vi "Loading Sequence.vi"(8 "Abort":bool, 9 "desired drop":dbl=8.0, 10 "Raised Tote Position":dbl=31.0, 11 "Button":bool) -> ()   [LabVIEW 2014]
uses:
  Loading States.ctl
  Robot Global Data.vi
  Desired Arm Position.vi
panel:
  out "Go all the way down":bool
  out "Wait for Unload":bool
  out "Lower Arms Slightly":bool
  out "Wait for Load":bool
  out "Raise Totes":bool
  out "Start + Wait for Totes":bool=TRUE
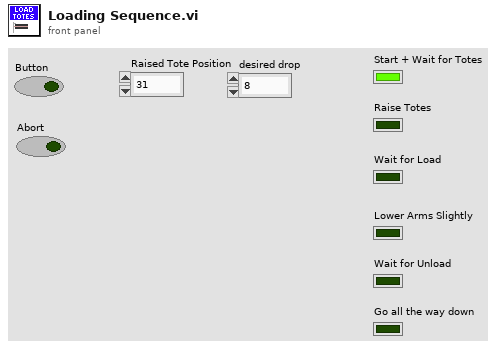
[diagram p1: front panel]
types:
  T1 = typedef "Loading States.ctl" = enum16{"Start+Wait for Totes", "Raise 2 Totes", "Wait for Loading", "Lower 2 Totes slightly", "Wait for Unload", "Go All the Way Down"}
  T2 = typedef "WPI_DigitalInputDevRef.ctl" = cluster{"DevStatus":errorcluster, "DIO Channel":T3, "Controller":T4}
  T3 = typedef "FPGA_DIOChannel.ctl" = enum8{"DIO 0", "DIO 1", "DIO 2", "DIO 3", "DIO 4", "DIO 5", "DIO 6", "DIO 7", "DIO 8", "DIO 9", "DIO MXP 0", "DIO MXP 1", "DIO MXP 2", "DIO MXP 3", "DIO MXP 4", "DIO MXP 5", "DIO MXP 6", "DIO MXP 7", "DIO MXP 8", "DIO MXP 9", "DIO MXP 10", "DIO MXP 11", "DIO MXP 12", "DIO MXP 13", "DIO MXP 14", "DIO MXP 15", "Invalid"}
  T4 = typedef "FPGA_TypedefDigitalModule.ctl" = enum16{"Controller 1"}
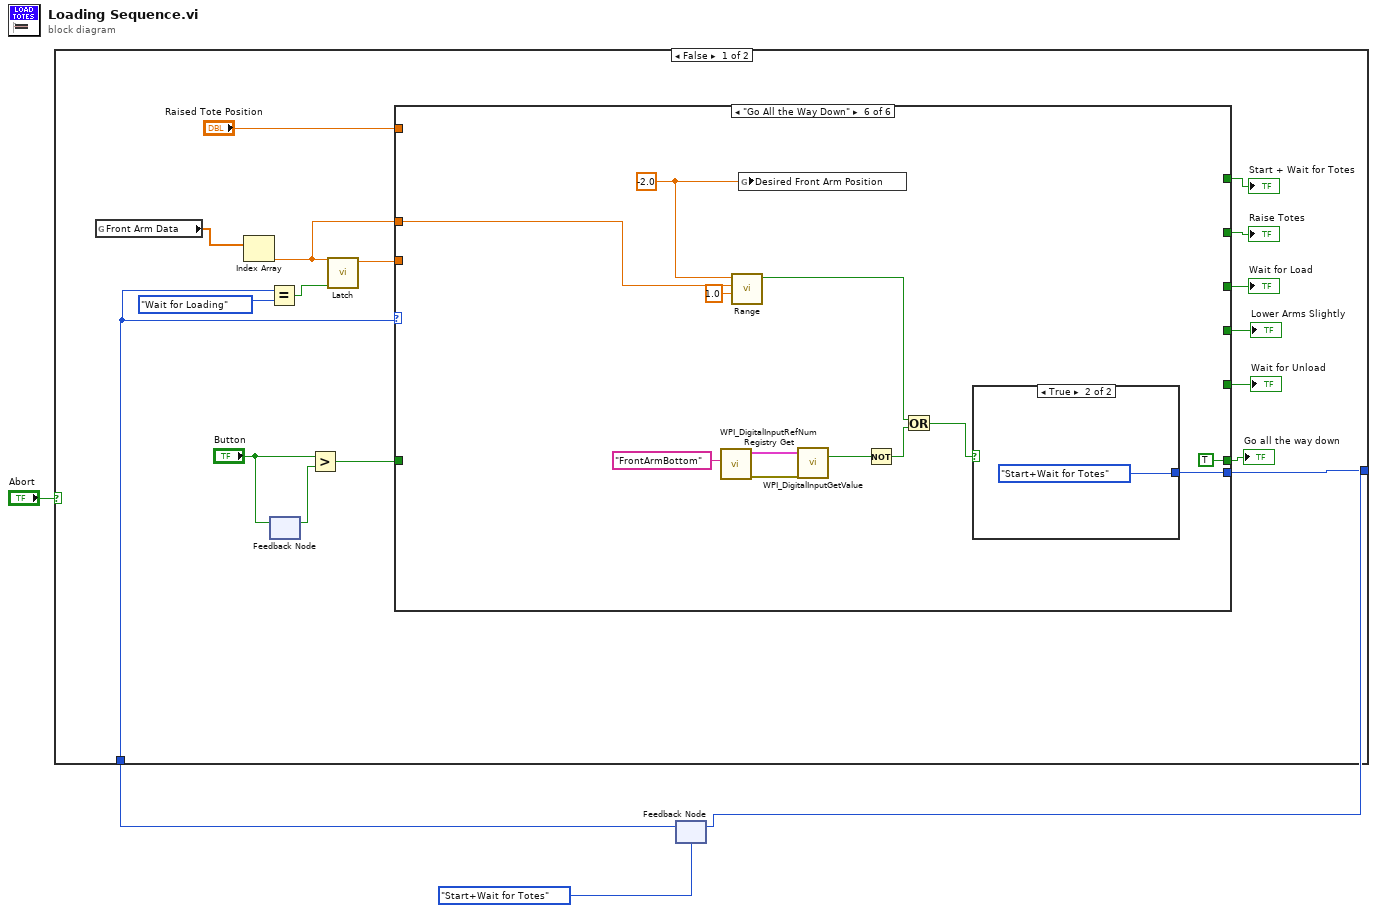
[diagram p0: block diagram]
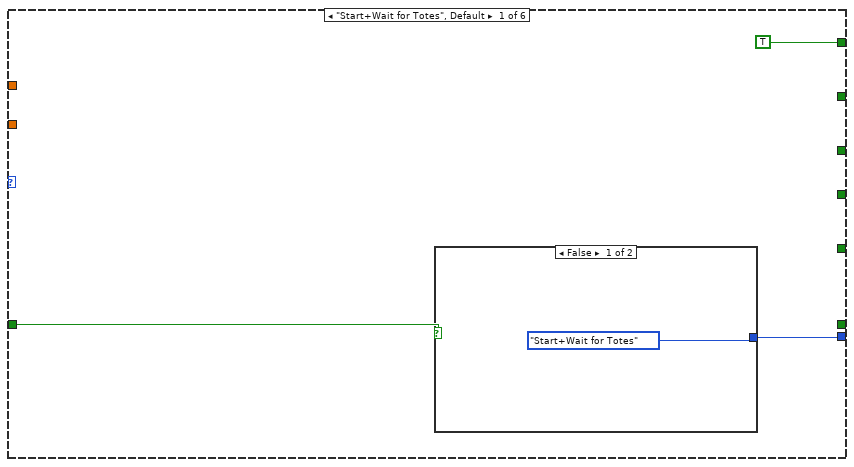
[diagram p2: hidden frame]
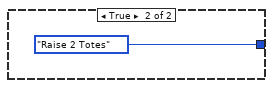
[diagram p3: hidden frame]
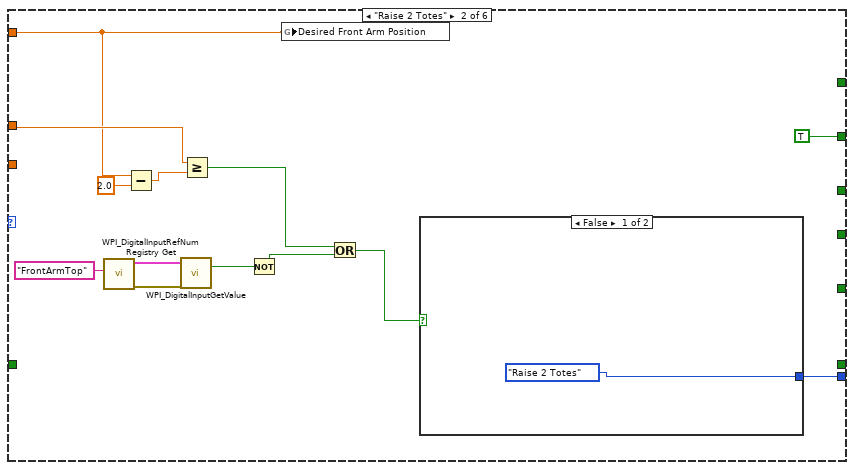
[diagram p4: hidden frame]
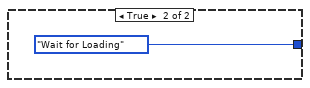
[diagram p5: hidden frame]
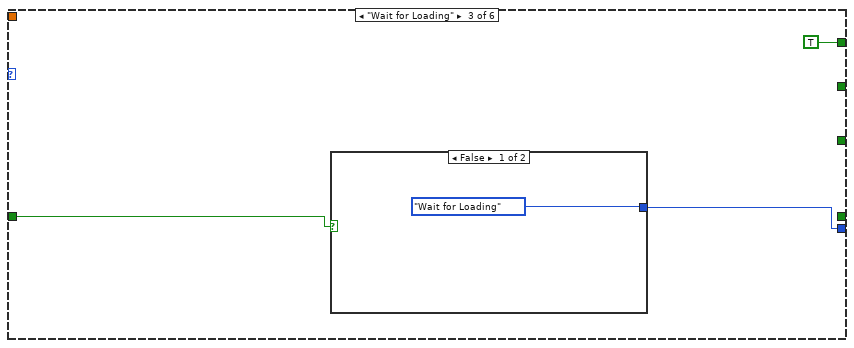
[diagram p6: hidden frame]
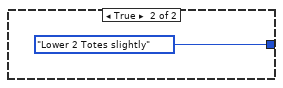
[diagram p7: hidden frame]
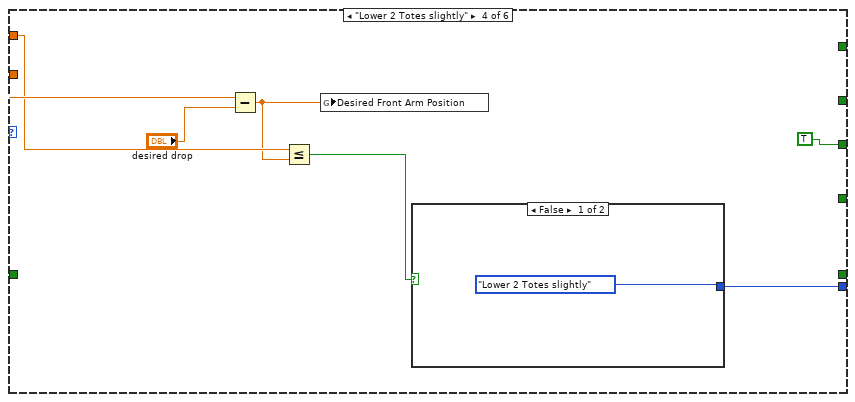
[diagram p8: hidden frame]
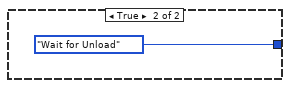
[diagram p9: hidden frame]
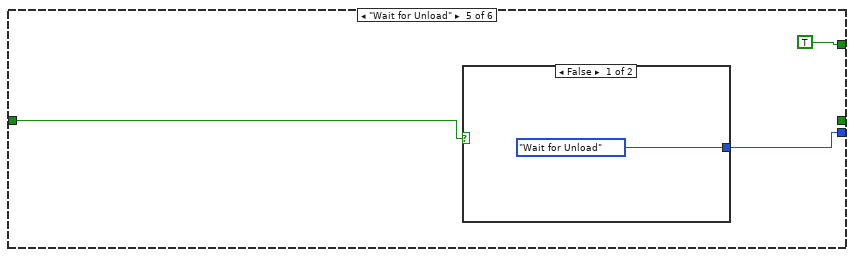
[diagram p10: hidden frame]
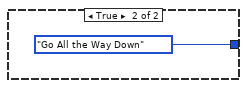
[diagram p11: hidden frame]
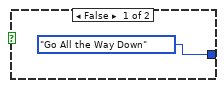
[diagram p12: hidden frame]
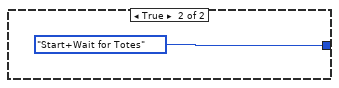
[diagram p13: hidden frame]
diagram:
  n1 = feedback #1(Loading_States."Start+Wait for Totes" ("Enum")) -> (w1:T1)
  n2 = case shown="False" "Abort" {
    tunnel: [w13 Loading_States."Start+Wait for Totes" ("Enum")] -> w2
    tunnel: w1 -> [w12 _]
    frame False {
      n3 = global read "Robot Global Data.vi" "Front Arm Data"() -> (w17:dbl[])
      n4 = Index Array(array=w17) -> (element=w5:dbl)  [unwired: 1 in]
      n5 = Equal?(x=w12, y=Loading_States."Wait for Loading" ("Enum")) -> (x = y?=w14:bool)
      n6 = feedback #2() -> (w20:bool)  [unwired: 1 in]
      n7 = feedback-in #2("Button") -> ()
      n8 = Greater?(x="Button", y=w20) -> (0:w18:bool)
      n9 = call "Latch.vi"("Reset"=w14, "Input"=w5) -> ("Output"=w16:dbl)  [unwired: 9 in]
      n10 = case shown="\"Go All the Way Down\"" w12 {
        tunnel: "Raised Tote Position" -> [_ w30 _ _ _ _]
        tunnel: w18 -> [w24 _ w44 _ w58 _]
        tunnel: [w23 w33 w43 w51 w57 w68] -> w13
        tunnel: w16 -> [_ _ _ w52 _ _]
        tunnel: [TRUE _ _ _ _ _] -> w11
        tunnel: [_ TRUE _ _ _ _] -> w10
        tunnel: [_ _ TRUE _ _ _] -> w9
        tunnel: [_ _ _ TRUE _ _] -> w8
        tunnel: [_ _ _ _ TRUE _] -> w7
        tunnel: [_ _ _ _ _ TRUE] -> w6
        tunnel: w5 -> [_ w31 _ w49 _ w65]
        frame "Start+Wait for Totes", Default {
          n11 = case shown="False" w24 {
            tunnel: [Loading_States."Start+Wait for Totes" ("Enum") Loading_States."Raise 2 Totes" ("Enum")] -> w23
            frame False {
            }
            frame True {
            }
          }
        }
        frame "Raise 2 Totes" {
          n12 = call <vilib>:"WPI_DigitalInputRefNum Registry Get.vi"("refnum name"="FrontArmTop") -> ("error out"=w38:errorcluster, "DigitalInputDevRef"=w37:T2)  [unwired: 9 in]
          n13 = Subtract(x=w30, y=2.0) -> (x-y=w28:dbl)
          n14 = call <vilib>:"WPI_DigitalInputGetValue.vi"("error in (no error)"=w38, "DigitalInputDevRef"=w37) -> ("Value"=w36:bool)  [unwired: 7 in, 2 out]
          n15 = Greater Or Equal?(x=w31, y=w28) -> (x >= y?=w27:bool)
          n16 = Not(x=w36) -> (.not. x?=w35:bool)
          n17 = global write "Desired Arm Position.vi" "Desired Front Arm Position"(w30) -> ()
          n18 = Or(x=w27, y=w35) -> (x .or. y?=w34:bool)
          n19 = case shown="False" w34 {
            tunnel: [Loading_States."Raise 2 Totes" ("Enum") Loading_States."Wait for Loading" ("Enum")] -> w33
            frame False {
            }
            frame True {
            }
          }
        }
        frame "Wait for Loading" {
          n20 = case shown="False" w44 {
            tunnel: [Loading_States."Wait for Loading" ("Enum") Loading_States."Lower 2 Totes slightly" ("Enum")] -> w43
            frame False {
            }
            frame True {
            }
          }
        }
        frame "Lower 2 Totes slightly" {
          n21 = Subtract(x=w52, y="desired drop") -> (x-y=w48:dbl)
          n22 = Less Or Equal?(x=w49, y=w48) -> (x <= y?=w47:bool)
          n23 = global write "Desired Arm Position.vi" "Desired Front Arm Position"(w48) -> ()
          n24 = case shown="False" w47 {
            tunnel: [Loading_States."Lower 2 Totes slightly" ("Enum") Loading_States."Wait for Unload" ("Enum")] -> w51
            frame False {
            }
            frame True {
            }
          }
        }
        frame "Wait for Unload" {
          n25 = case shown="False" w58 {
            tunnel: [Loading_States."Wait for Unload" ("Enum") Loading_States."Go All the Way Down" ("Enum")] -> w57
            frame False {
            }
            frame True {
            }
          }
        }
        frame "Go All the Way Down" {
          w64 = -2.0 ("Desired Front Arm Position")
          n26 = call <vilib>:"WPI_DigitalInputRefNum Registry Get.vi"("refnum name"="FrontArmBottom") -> ("error out"=w71:errorcluster, "DigitalInputDevRef"=w70:T2)  [unwired: 9 in]
          n27 = call "Range.vi"("Range"=1.0, "Input"=w65, "In Range of"=w64) -> ("In Range?"=w62:bool)  [unwired: 8 in]
          n28 = global write "Desired Arm Position.vi" "Desired Front Arm Position"(w64) -> ()
          n29 = call <vilib>:"WPI_DigitalInputGetValue.vi"("error in (no error)"=w71, "DigitalInputDevRef"=w70) -> ("Value"=w69:bool)  [unwired: 7 in, 2 out]
          n30 = Not(x=w69) -> (.not. x?=w66:bool)
          n31 = Or(x=w62, y=w66) -> (x .or. y?=w61:bool)
          n32 = case shown="True" w61 {
            tunnel: [Loading_States."Go All the Way Down" ("Enum") Loading_States."Start+Wait for Totes" ("Enum")] -> w68
            frame False {
            }
            frame True {
            }
          }
        }
      }
      "Lower Arms Slightly" <- w8
      "Start + Wait for Totes" <- w11
      "Raise Totes" <- w10
      "Wait for Load" <- w9
      "Wait for Unload" <- w7
      "Go all the way down" <- w6
    }
    frame True {
    }
  }
  n33 = feedback-in #1(w2) -> ()
